vi "Single_measurement.vi"(0 "LockIn VISA":refnum<visa-resource-name>="GPIB0::9::INSTR", 1 "LockIn VISA 2":refnum<visa-resource-name>="GPIB0::4::INSTR", 2 "Detecror signal":refnum<k21>, 3 "Hall-sensor calibration (mV/mT)":dbl=14.0 format="%0.2f", 5 "DAQ?":bool, 6 "Lakeshore VISA":refnum<visa-resource-name>="GPIB0::12::INSTR", 7 "seconds since 1Jan1904":timestamp, 8 "Keithly or myDAQ":bool=TRUE, 9 "Magnetic Background":dbl, 10 "Keithley VISA 2":refnum<visa-resource-name>="GPIB0::20::INSTR", 11 "error in (no error)":errorcluster, 12 "Dual Lockin":bool, 13 "Pt1000":refnum<k21>, 14 "Hall":refnum<k21>) -> (4 "Measurement":T1={"Elapsed Time (s)"=0.0, "Hall-sensor (mT)"=0.0, "LockIn A"=[1.33515e-05, 1.14442e-05, 1.90736e-05, 41.634], "LockIn B"=[1.33515e-05, 1.14442e-05, 1.90736e-05, 41.634], "Dc Intensity (V)"=0.0, "Temperature (K)"=0.0}, 15 "error out":errorcluster)   [LabVIEW 2017]
uses:
  <vilib>/DAQmx/read.llb/DAQmx Read (Analog DBL 1Chan 1Samp).vi
  <vilib>/DAQmx/read.llb/DAQmx Read (Analog 1D DBL 1Chan NSamp).vi
  <vilib>/Analysis/baseanly.llb/Mean (DBL).vi
  <vilib>/DAQmx/read.llb/DAQmx Read (Analog 1D DBL NChan 1Samp).vi
  <vilib>/DAQmx/miscellaneous.llb/DAQmx Fill In Error Info.vi
  <vilib>/Analysis/NI_AALBase.lvlib
panel:
  out "Temperature":dbl
  in  "Lakeshore?":bool=TRUE
  out "Rt":dbl
  in  "Plus Resistance":dbl=100.0
  out "read buffer 2":string="1.33515e-005,1.14442e-005,1.90736e-005,41.634\n"
  out "read buffer":string="1.33515e-005,1.14442e-005,1.90736e-005,41.634\n"
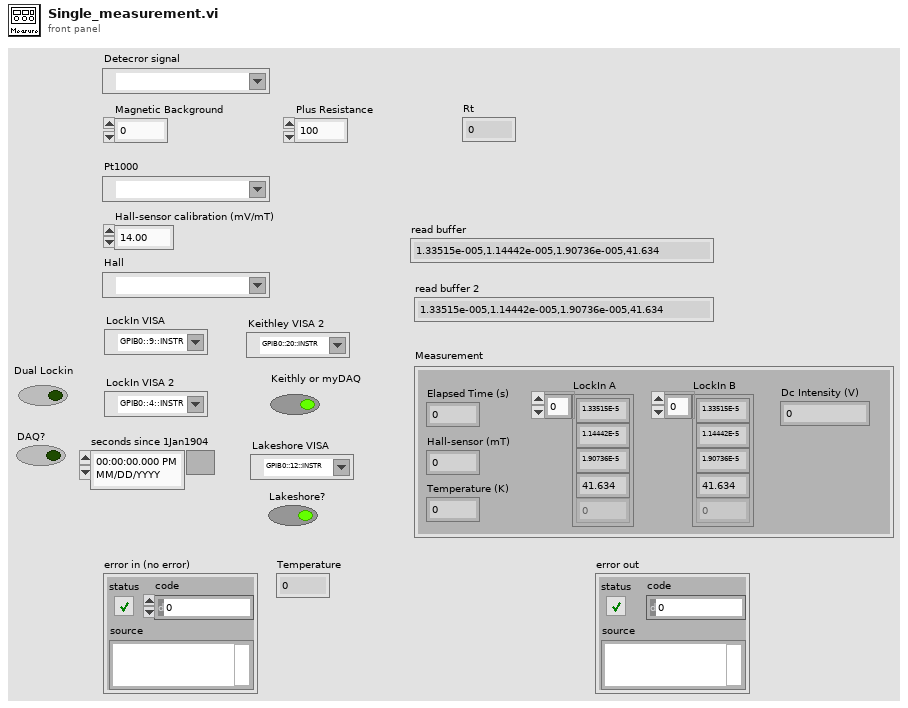
[diagram p1: front panel]
types:
  T1 = cluster{"Elapsed Time (s)":dbl, "Hall-sensor (mT)":dbl, "LockIn A":dbl[], "LockIn B":dbl[], "Dc Intensity (V)":dbl, "Temperature (K)":dbl}
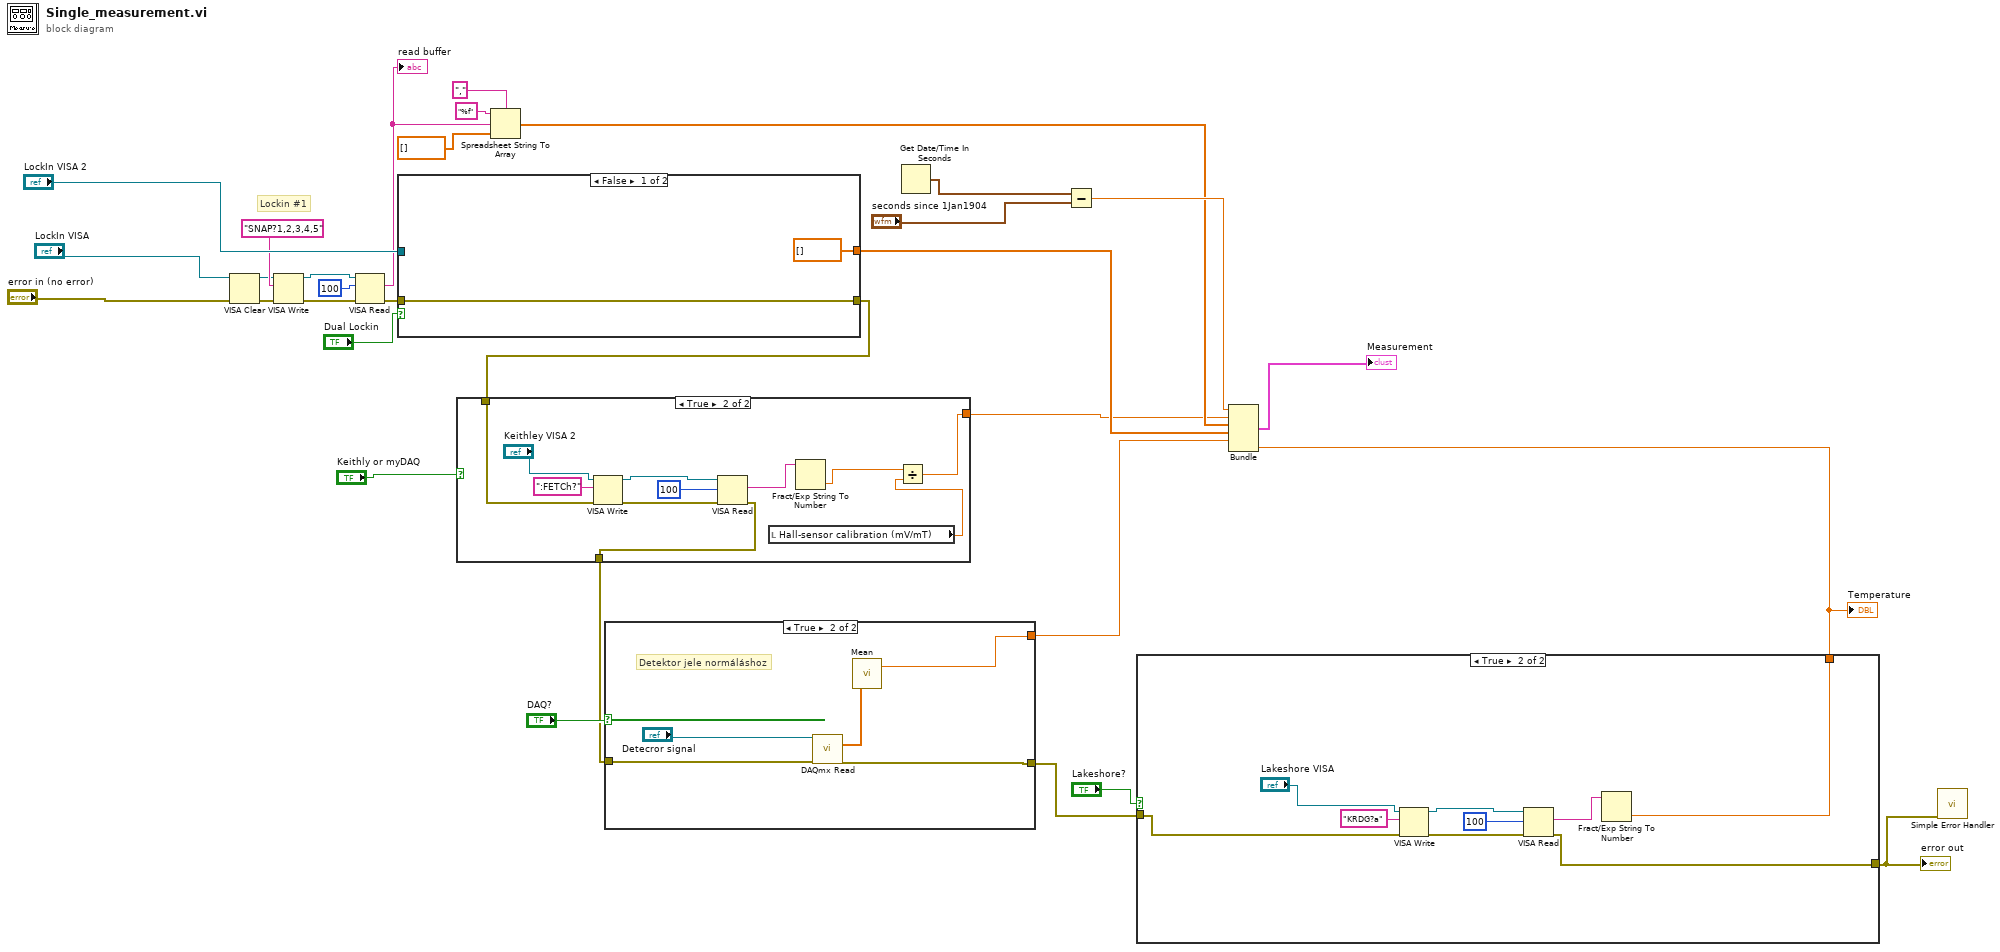
[diagram p0: block diagram]
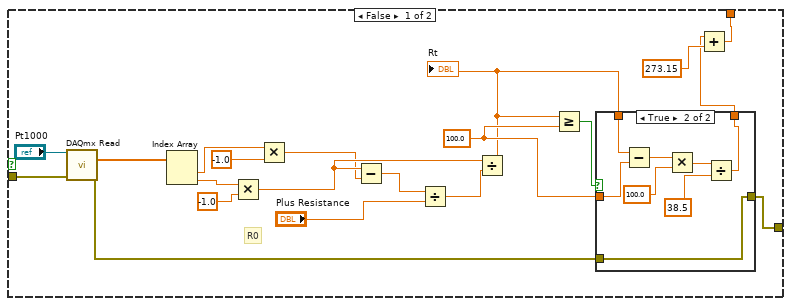
[diagram p2: hidden frame]
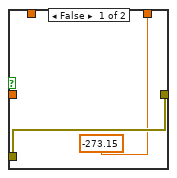
[diagram p3: hidden frame]
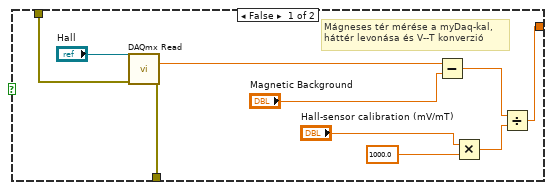
[diagram p4: hidden frame]
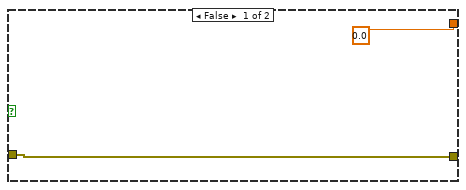
[diagram p5: hidden frame]
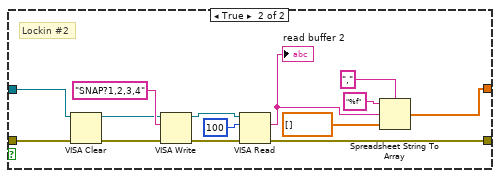
[diagram p6: hidden frame]
diagram:
  # "Lockin #1"
  n1 = VISA Clear(VISA resource name="LockIn VISA", error in (no error)="error in (no error)") -> (VISA resource name out=w12:refnum<visa-resource-name>, error out=w14:errorcluster)
  n2 = VISA Write(VISA resource name=w12, write buffer="SNAP?1,2,3,4,5" ("data"), error in (no error)=w14) -> (VISA resource name out=w26:refnum<visa-resource-name>, error out=w24:errorcluster)  [unwired: 1 out]
  n3 = VISA Read(VISA resource name=w26, byte count=100, error in (no error)=w24) -> (read buffer=w22:string, error out=w15:errorcluster)  [unwired: 2 out]
  "read buffer" <- w22
  n4 = case shown="False" "Dual Lockin" {
    tunnel: w15 -> [w33 w37]
    tunnel: "LockIn VISA 2" -> [_ w35]
    tunnel: [w33 w39] -> w8
    tunnel: [dbl[] [] w38] -> w17
    frame False {
    }
    frame True {
      # "Lockin #2"
      n5 = VISA Clear(VISA resource name=w35, error in (no error)=w37) -> (VISA resource name out=w34:refnum<visa-resource-name>, error out=w36:errorcluster)
      n6 = VISA Write(VISA resource name=w34, write buffer="SNAP?1,2,3,4" ("data"), error in (no error)=w36) -> (VISA resource name out=w47:refnum<visa-resource-name>, error out=w45:errorcluster)  [unwired: 1 out]
      n7 = VISA Read(VISA resource name=w47, byte count=100, error in (no error)=w45) -> (read buffer=w43:string, error out=w39:errorcluster)  [unwired: 2 out]
      "read buffer 2" <- w43
      n8 = Spreadsheet String To Array(delimiter (Tab)=",", format string="%f", spreadsheet string=w43, array type (2D Dbl)=dbl[] []) -> (array=w38:dbl[])
    }
  }
  n9 = case shown="True" "Keithly or myDAQ" {
    tunnel: [w57 w59] -> w11
    tunnel: w8 -> [w49 w62]
    tunnel: [w48 w61] -> w7
    frame False {
      # "Mágneses tér mérése a myDaq-kal,\nháttér levonása és V--T konverzió"
      n10 = call-poly <vilib>:"DAQmx Read.vi"("task/channels in"="Hall", "error in"=w49) -> ("data"=w55:dbl, "error out"=w48:errorcluster)  [unwired: 11 in, 1 out]
      n11 = Subtract(x=w55, y="Magnetic Background") -> (x-y=w56:dbl)
      n12 = Multiply(x="Hall-sensor calibration (mV/mT)", y=1000.0) -> (x*y=w53:dbl)
      n13 = Divide(x=w56, y=w53) -> (x/y=w57:dbl)
    }
    frame True {
      n14 = VISA Write(VISA resource name="Keithley VISA 2", write buffer=":FETCh?" ("data"), error in (no error)=w62) -> (VISA resource name out=w66:refnum<visa-resource-name>, error out=w65:errorcluster)  [unwired: 1 out]
      n15 = VISA Read(VISA resource name=w66, byte count=100, error in (no error)=w65) -> (read buffer=w68:string, error out=w61:errorcluster)  [unwired: 2 out]
      n16 = local read "Hall-sensor calibration (mV/mT)"() -> (w60:dbl)
      n17 = Fract/Exp String To Number(string=w68) -> (number=w58:dbl)  [unwired: 3 in, 1 out]
      n18 = Divide(x=w58, y=w60) -> (x/y=w59:dbl)
    }
  }
  n19 = Spreadsheet String To Array(delimiter (Tab)=",", format string="%f", spreadsheet string=w22, array type (2D Dbl)=dbl[] []) -> (array=w18:dbl[])
  n20 = case shown="True" "DAQ?" {
    tunnel: [w70 w73] -> w6
    tunnel: w7 -> [w70 w71]
    tunnel: [0.0 ("mean") w74] -> w4
    frame False {
    }
    frame True {
      # "Detektor jele normáláshoz"
      n21 = call-poly <vilib>:"DAQmx Read.vi"("task/channels in"="Detecror signal", "error in"=w71) -> ("data"=w75:dbl[], "error out"=w73:errorcluster)  [unwired: 11 in, 1 out]
      n22 = call-poly <vilib>:"Mean.vi"("X"=w75) -> ("mean"=w74:dbl)  [unwired: 1 out]
    }
  }
  n23 = Get Date/Time In Seconds() -> (seconds since 1Jan1904=w29:timestamp)
  n24 = Subtract(x=w29, y="seconds since 1Jan1904") -> (x-y=w31:dbl)
  n25 = case shown="True" "Lakeshore?" {
    tunnel: w6 -> [w86 w109]
    tunnel: [w85 w108] -> w5
    tunnel: [w76 w106] -> w2
    frame False {
      w94 = 100.0 ("y")
      # "R0"
      n26 = call-poly <vilib>:"DAQmx Read.vi"("task/channels in"="Pt1000", "error in"=w86) -> ("data"=w90:dbl[], "error out"=w88:errorcluster)  [unwired: 11 in, 1 out]
      n27 = Index Array(array=w90) -> (element #1=w83:dbl, element #2=w84:dbl)  [unwired: 2 in]
      n28 = Multiply(x=w84, y=-1.0) -> (x*y=w80:dbl)
      n29 = Multiply(x=w83, y=-1.0) -> (x*y=w79:dbl)
      n30 = Subtract(x=w80, y=w79) -> (x-y=w93:dbl)
      n31 = Divide(x=w93, y="Plus Resistance") -> (x/y=w92:dbl)
      n32 = Divide(x=w80, y=w92) -> (x/y=w89:dbl)
      "Rt" <- w89
      n33 = Greater Or Equal?(x=w89, y=w94) -> (x >= y?=w95:bool)
      n34 = case shown="True" w95 {
        tunnel: w88 -> [w97 w105]
        tunnel: [w97 w105] -> w85
        tunnel: w89 -> [_ w104]
        tunnel: w94 -> [_ w103]
        tunnel: [-273.15 w98] -> w77
        frame False {
        }
        frame True {
          n35 = Subtract(x=w104, y=w103) -> (x-y=w100:dbl)
          n36 = Multiply(x=w100, y=100.0) -> (x*y=w102:dbl)
          n37 = Divide(x=w102, y=38.5) -> (x/y=w98:dbl)
        }
      }
      n38 = Add(x=w77, y=273.15) -> (x+y=w76:dbl)
    }
    frame True {
      n39 = VISA Write(VISA resource name="Lakeshore VISA", write buffer="KRDG?a" ("data"), error in (no error)=w109) -> (VISA resource name out=w113:refnum<visa-resource-name>, error out=w112:errorcluster)  [unwired: 1 out]
      n40 = VISA Read(VISA resource name=w113, byte count=100, error in (no error)=w112) -> (read buffer=w114:string, error out=w108:errorcluster)  [unwired: 2 out]
      n41 = Fract/Exp String To Number(string=w114) -> (number=w106:dbl)  [unwired: 3 in, 1 out]
    }
  }
  "error out" <- w5
  "Temperature" <- w2
  n42 = Bundle(w31, w11, w18, w17, "mean"=w4, w2) -> (→"Measurement":cluster{dbl, dbl, dbl[], dbl[], "mean":dbl, dbl})  [unwired: 1 in]
  n43 = call <vilib>:"Simple Error Handler.vi"("error in (no error)"=w5) -> ()  [unwired: 4 in, 5 out]
